vi "Draw.vi"(8 "error in (no error)":errorcluster, 11 "Layered Shape in":refnum<class "Layered Shape.lvclass">) -> (0 "error out":errorcluster, 2 "Picture":picture, 3 "Layered Shape out":refnum<class "Layered Shape.lvclass">)   [LabVIEW 2015, in "LV Image Editor Framework.lvlib" / "Layered Shape.lvclass"]
uses:
  Layered Shape.lvclass
  Shape/Shape.lvclass
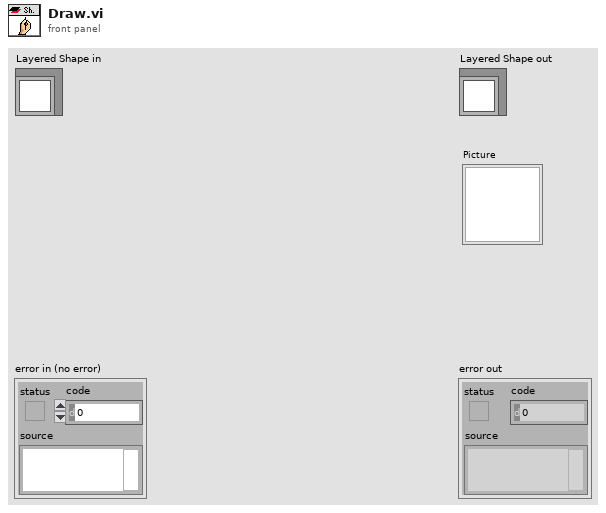
[diagram p1: front panel]
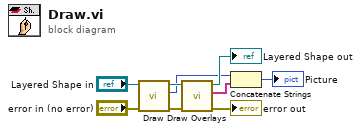
[diagram p0: block diagram]
diagram:
  n1 = call-parent "Draw.vi"("error in (no error)"="error in (no error)", "Shape in"="Layered Shape in") -> ("error out"=w5:errorcluster, "Picture"=w2:picture, "Shape out"=w7:refnum<class "Layered Shape.lvclass">)  [unwired: 7 in]
  n2 = call-dynamic "Draw Overlays.vi"("error in (no error)"=w5, "Rectangle in"=w7) -> ("error out"=→"error out":errorcluster, "Overlays"=w3:string[], "Rectangle out"=→"Layered Shape out":refnum<class "Layered Shape.lvclass">)  [unwired: 7 in]
  n3 = Concatenate Strings(w2, w3) -> (→"Picture":picture)
